vi "GT Enable Gantry.vi"(6 "slaveKp":dbl, 7 "masterKp":dbl, 8 "error in (no error)":errorcluster caption="错误输入（无错误）", 9 "gantrySlave":i16, 10 "gantryMaster":i16, 11 "cardNum":i16) -> (0 "error out":errorcluster caption="错误输出", 3 "function return":i16)   [LabVIEW 2014, in "gts.lvlib"]
doc: "GT_API GT_EnableGantry(short cardNum,short gantryMaster,short gantrySlave,double masterKp,double slaveKp);"
uses:
  gts.lvlib
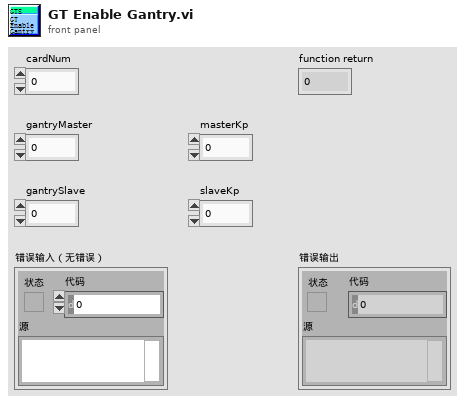
[diagram p1: front panel]
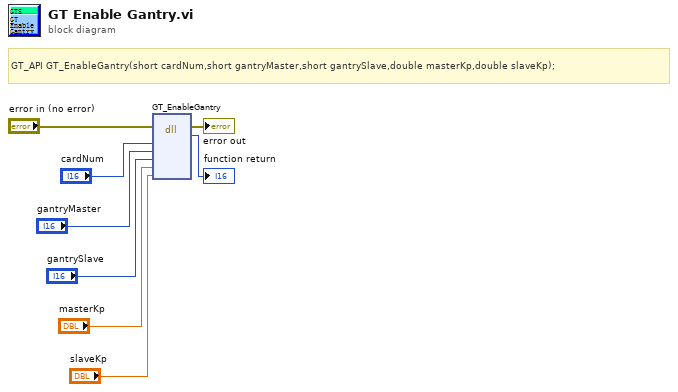
[diagram p0: block diagram]
diagram:
  # "GT_API GT_EnableGantry(short cardNum,short gantryMaster,short gantrySlave,double masterKp,double slaveKp);"
  n1 = dll-call lib="PTH2habs D固高科技资料GTS控制卡GTS卡18年上半年资料dllVC32bit\nmulti_cardgts.*" fn="GT_EnableGantry"(error in="error in (no error)", "cardNum"="cardNum", "gantryMaster"="gantryMaster", "gantrySlave"="gantrySlave", "masterKp"="masterKp", "slaveKp"="slaveKp") -> (error out=→"error out":errorcluster, →"function return":i16)  [unwired: 7 in, 1 out]
